vi "ApplyKalman.vi"(4 "Variables Array":T3, 5 "Init State":T2, 8 "Sample Interval (sec)":dbl, 9 "Frm Indx":dbl, 10 "P_n_1":T1, 11 "Dpp Array":dbl[](array[numeric])) -> (1 "Trend":dbl, 2 "P_n_n_1":T1, 3 "State Array Out":T2)   [LabVIEW 2012]
uses:
  <vilib>/Analysis/Matrix/Datatypes/RealMatrix.ctl
  <vilib>/Analysis/Matrix/NI_Matrix.lvlib
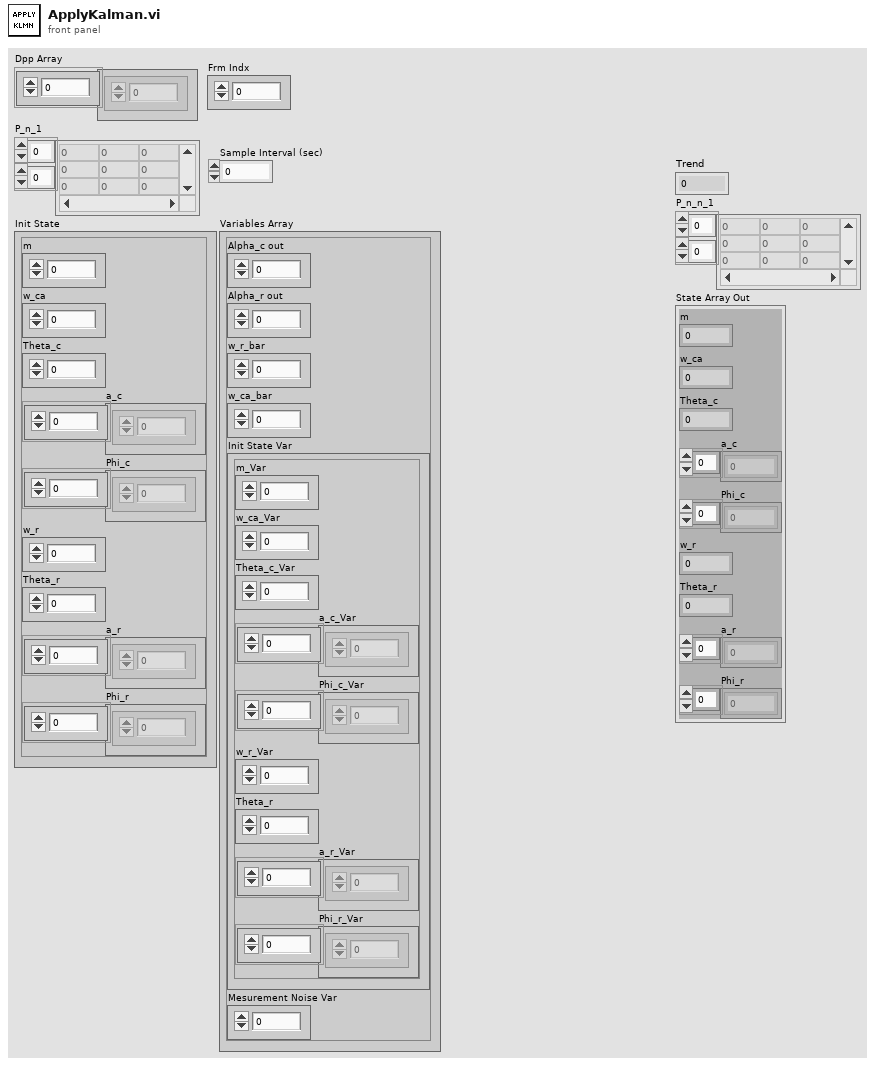
[diagram p1: front panel]
types:
  T1 = typedef "NI_Matrix.lvlib/RealMatrix.ctl" = dbl[][]
  T2 = cluster{"m":dbl, "w_ca":dbl, "Theta_c":dbl, "a_c":dbl[], "Phi_c":dbl[], "w_r":dbl, "Theta_r":dbl, "a_r":dbl[], "Phi_r":dbl[]}
  T3 = cluster{"Alpha_c out":dbl, "Alpha_r out":dbl, "w_r_bar":dbl, "w_ca_bar":dbl, "Init State Var":cluster{"m_Var":dbl, "w_ca_Var":dbl, "Theta_c_Var":dbl, "a_c_Var":dbl[], "Phi_c_Var":dbl[], "w_r_Var":dbl, "Theta_r":dbl, "a_r_Var":dbl[], "Phi_r_Var":dbl[]}, "Mesurement Noise Var":dbl}
  T4 = cluster{"m_Var":dbl, "w_ca_Var":dbl, "Theta_c_Var":dbl, "a_c_Var":dbl[], "Phi_c_Var":dbl[], "w_r_Var":dbl, "Theta_r":dbl, "a_r_Var":dbl[], "Phi_r_Var":dbl[]}
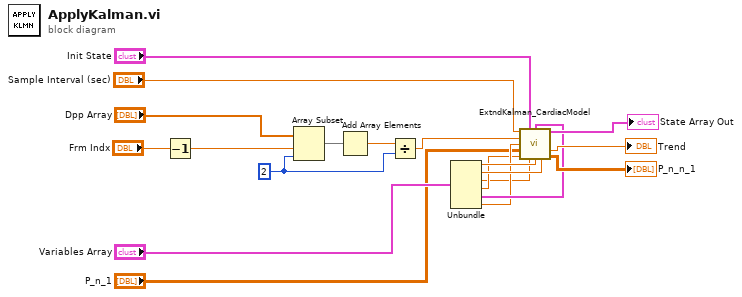
[diagram p0: block diagram]
diagram:
  w5 = 2 ("length")
  n1 = Decrement(x="Frm Indx") -> (x-1=w16:dbl)
  n2 = Array Subset(array="Dpp Array", index=w16, length=w5) -> (w14:dbl[])
  n3 = Add Array Elements(numeric array=w14) -> (sum=w6:dbl)
  n4 = Divide(x=w6, y=w5) -> (x/y=w7:dbl)
  n5 = Unbundle("Variables Array") -> ("Alpha_c out"=w12:dbl, "Alpha_r out"=w11:dbl, "w_r_bar"=w8:dbl, "w_ca_bar"=w9:dbl, "Init State Var"=w13:T4, "Mesurement Noise Var"=w10:dbl)
  n6 = call "ExtndKalman_CardiacModel.vi"("Sample Interval (sec)"="Sample Interval (sec)", "State_n_n"="Init State", "State_n_n Var"=w13, "y_n (hemodynamic value)"=w7, "Noise Var (r)"=w10, "P_n_1"="P_n_1", "w_bar_ca"=w9, "w_bar_r"=w8, "Alpha_c"=w12, "Alpha_r"=w11) -> ("Output State"=→"State Array Out":T2, "Trend"=→"Trend":dbl, "P_n_n_1"=→"P_n_n_1":T1)  [unwired: 3 in]
